vi "Teleop.vi"(10 "Match Info":T1={"Autonomous Elapsed Seconds"=0.0, "TeleOp Elapsed Seconds"=0.0, "Disabled Elapsed Seconds"=0.0, "Visited Autonomous"=FALSE, "Visited TeleOp"=FALSE, "Visited Disabled"=FALSE, "Autonomous Settings"={"Autonomous Style"=enum."Independent", "VI Refnum"=refnum}}, 11 "Call Context":T2) -> ()   [LabVIEW 2014]
doc: "This VI is called for each TeleOp packet received from the DS where the robot is not disabled. It is often used to read from the joysticks and update I/O or to update setpoints for timed control loops. It should complete and return within 20 milliseconds or it may miss DS packets."
uses:
  <vilib>/Rock Robotics/WPI/DriverStation/WPI_DriverStationDerivedRobotMode.ctl
  <vilib>/Rock Robotics/WPI/DriverStation/WPI_DriverStationMatch Info.ctl
  <vilib>/Rock Robotics/Network Tables/SD Read Boolean.vi
  <vilib>/Rock Robotics/Network Tables/SD Read Number.vi
  <vilib>/Rock Robotics/Network Tables/SD Write Numeric Array.vi
  1756_Code/General_VI/Global Var.vi
  <vilib>/Rock Robotics/Network Tables/SD Write Boolean Array.vi
panel:
  out "Sample Slider 0":dbl(slide) scale=0.0..5.0
  out "Sample Boolean 1":bool
  out "Sample Boolean 0":bool
  # "e"
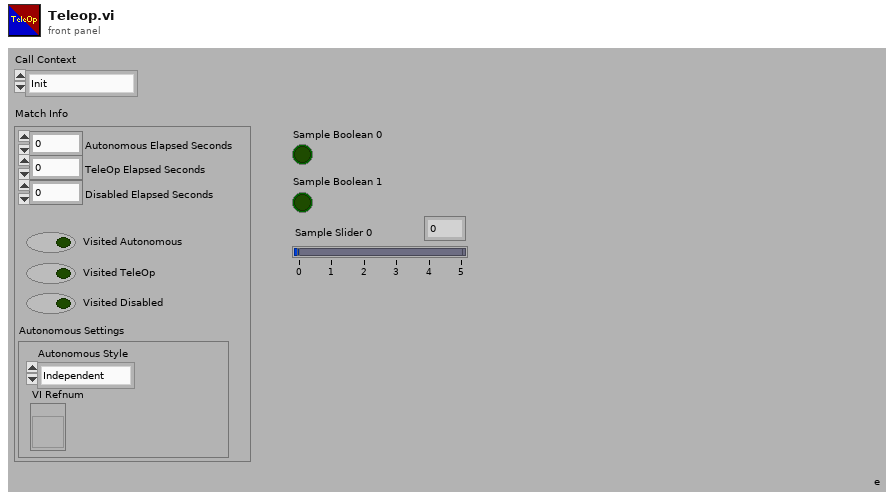
[diagram p1: front panel]
types:
  T1 = typedef "WPI_DriverStationMatch Info.ctl" = cluster{"Autonomous Elapsed Seconds":dbl, "TeleOp Elapsed Seconds":dbl, "Disabled Elapsed Seconds":dbl, "Visited Autonomous":bool, "Visited TeleOp":bool, "Visited Disabled":bool, "Autonomous Settings":cluster{"Autonomous Style":enum16{"Iterative", "Independent"}, "VI Refnum":refnum<vi>}}
  T2 = typedef "WPI_DriverStationDerivedRobotMode.ctl" = enum16{"Init", "Execute", "Stop"}
  T3 = typedef "WPI_JoystickDevRef.ctl" = cluster{"Device":T4}
  T4 = typedef "WPI_JoystickDeviceEnum.ctl" = enum16{"USB 0", "USB 1", "USB 2", "USB 3", "USB 4", "USB 5"}
  T5 = typedef "WPI_RobotDriveDevRef.ctl" = cluster{"DevStatus":errorcluster, "Motors[]":T6[], "Square Inputs":bool, "Max Output":dbl}
  T6 = typedef "WPI_MotorControlDeviceRef.ctl" = cluster{"DeviceStatus":errorcluster, "Type":T7, "PWM":cluster{"Controller":T8, "PWM Channel":T9, "DeadBand":T10}, "CAN":cluster{"Device Number":u8, "Control Mode":T11, "Semaphore":T12, "Max Vout":dbl, "TalonSRX Control Mode":T13}, "Invert":bool, "TransformRef":T14, "InvTransformRef":T14}
  T7 = typedef "WPI_MotorControlType.ctl" = enum16{"PWM", "CAN", "CANTalonSRX"}
  T8 = typedef "FPGA_TypedefDigitalModule.ctl" = enum16{"Controller 1"}
  T9 = typedef "FPGA_DIOPWMChannel.ctl" = enum8{"PWM 0", "PWM 1", "PWM 2", "PWM 3", "PWM 4", "PWM 5", "PWM 6", "PWM 7", "PWM 8", "PWM 9", "PWM MXP 0", "PWM MXP 1", "PWM MXP 2", "PWM MXP 3", "PWM MXP 4", "PWM MXP 5", "PWM MXP 6", "PWM MXP 7", "PWM MXP 8", "PWM MXP 9", "Invalid"}
  T10 = typedef "WPI_PWMDeadband.ctl" = cluster{"Name":string, "maxPositivePwm":i32, "minPositivePwm":i32, "centerPwm":i32, "maxNegativePwm":i32, "minNegativePwm":i32, "angularRange":u16}
  T11 = typedef "WPI_CANJaguar_ControlMode.ctl" = enum8{"Percent VBus", "Current", "Speed", "Position", "Voltage"}
  T12 = typedef "Semaphore RefNum" = refnum<k1>
  T13 = typedef "WPI_CANTalonSRX_APIControlMode.ctl" = enum8{"Percent VBus", "Speed", "Position", "Slave", "Unchanged / Invalid"}
  T14 = typedef "WPI_PWMTransform_ConPane.ctl" = refnum<vi>
  T15 = typedef "WPI_EncoderDevRef.ctl" = cluster{"DevStatus":errorcluster, "EncoderIndex":T16, "CounterIndex":T17, "DistancePerCount":dbl, "Decoding Type":T18}
  T16 = typedef "FPGA_EncoderIdx.ctl" = enum8{"Enc 0", "Enc 1", "Enc 2", "Enc 3", "Enc 4", "Enc 5", "Enc 6", "Enc 7", "Invalid"}
  T17 = typedef "FPGA_CounterCtrSystemIndex.ctl" = enum8{"Ctr 0", "Ctr 1", "Ctr 2", "Ctr 3", "Ctr 4", "Ctr 5", "Ctr 6", "Ctr 7", "Invalid"}
  T18 = typedef "WPI_EncoderType.ctl" = enum16{"1x", "2x", "4x"}
  T19 = typedef "WPI_SwitchDevRef.ctl" = cluster{"DevStatus":errorcluster, "DIO Channel":T20, "Controller":T8, "CntIndex":T17, "Normally Closed":bool}
  T20 = typedef "FPGA_DIOChannel.ctl" = enum8{"DIO 0", "DIO 1", "DIO 2", "DIO 3", "DIO 4", "DIO 5", "DIO 6", "DIO 7", "DIO 8", "DIO 9", "DIO MXP 0", "DIO MXP 1", "DIO MXP 2", "DIO MXP 3", "DIO MXP 4", "DIO MXP 5", "DIO MXP 6", "DIO MXP 7", "DIO MXP 8", "DIO MXP 9", "DIO MXP 10", "DIO MXP 11", "DIO MXP 12", "DIO MXP 13", "DIO MXP 14", "DIO MXP 15", "Invalid"}
  T21 = typedef "WPI_AnalogChannelDevRef.ctl" = cluster{"DevStatus":errorcluster, "Controller":T22, "Analog Channel":T23}
  T22 = typedef "FPGA_TypedefAnalogModule.ctl" = enum16{"Controller 1"}
  T23 = typedef "FPGA_AIChannel.ctl" = enum8{"AI 0", "AI 1", "AI 2", "AI 3", "AI MXP 0", "AI MXP 1", "AI MXP 2", "AI MXP 3", "Invalid"}
  T24 = typedef "IMUDevRef.ctl" = cluster{"DevStatus":errorcluster, "Gyro Address":u8, "Gyro Range":u8, "Mean Rates":cluster{"Xmo":dbl, "Ymo":dbl, "Zmo":dbl}, "StdDev Rates":cluster{"Xsdo":dbl, "Ysdo":dbl, "Zsdo":dbl}, "Fast":bool, "Reset":bool, "Accel Address":u8, "Accel Range":u8, "Accel Scale":cluster{"Xscale":dbl, "Yscale":dbl, "Zscale":dbl}, "Mag Address":u8, "Mag Range":u8, "G Sense":bool, "A Sense":bool, "M Sense":bool, "Accel Offset":cluster{"Xzero":dbl, "Yzero":dbl, "Zzero":dbl}, "Motion Thresh":dbl, "Mag Scale":cluster{"Xscale":dbl, "Yscale":dbl, "Zscale":dbl}, "Mag Offset":cluster{"Xzero":dbl, "Yzero":dbl, "Zzero":dbl}, "I2C Bus":T25, "Handle":i32, "Controller":T8, "Anomaly Thresh":dbl, "Local Mag":dbl}
  T25 = typedef "i2c_bus.ctl" = enum16{"I2C On-Board", "I2C MXP", "Invalid"}
  T26 = typedef "WPI_CompressorDevRef.ctl" = cluster{"DevStatus":errorcluster, "Pneumatics Control Module":u8}
  T27 = typedef "WPI_SolenoidDevRef.ctl" = cluster{"DevStatus":errorcluster, "Pneumatics Control Module":u8, "Forward Solenoid Channel":T28, "Reverse Solenoid Channel":T28}
  T28 = typedef "WPI_SolenoidChannel.ctl" = enum8{"Solenoid 0", "Solenoid 1", "Solenoid 2", "Solenoid 3", "Solenoid 4", "Solenoid 5", "Solenoid 6", "Solenoid 7", "Invalid"}
  T29 = cluster{"Joystick":cluster{"Drive_Joystick":T3, "Imp_Joystick":T3}, "Motor":cluster{"Left and Right Motors":T5, "Left_Intake":T6, "Right_Intake":T6, "Elevator_Lift":T6, "Elevator_Arm_Left":T6, "Elevator_Arm_Right":T6}, "Encoder":cluster{"Left_Drive_Speed":T15, "Auto_2_Tote":T19, "Auto_Cans":T19, "Auto_Cans_Delay":T19}, "Analog":cluster{"Tote_Detect_1":T21, "Tote_Detect_2":T21, "Ele_Pos_Yoyo":T21, "Auto_Switch":T21}, "IMU_Reft_Num":T24, "Pneumatics":cluster{"Compressor":T26, "Arm_Sol":T27, "Infeed_Pneu":T27, "Can_Tip_Flip":T27, "Can_Tip_Arm":T27, "Can_Door_Arm":T27, "Arm_Sol_Ext":T27}}
  T30 = cluster{"Left_Trigger":dbl, "Right_Trigger ":dbl, "Left_X":dbl, "Left_Y":dbl, "Right_X":dbl, "Right_Y":dbl}
  T31 = cluster{"A":bool, "B":bool, "X":bool, " Y":bool, "LB":bool, " RB":bool, "Left_Thumb_Button":bool, "Right_Thumb_Button":bool, "Back":bool, "Start":bool}
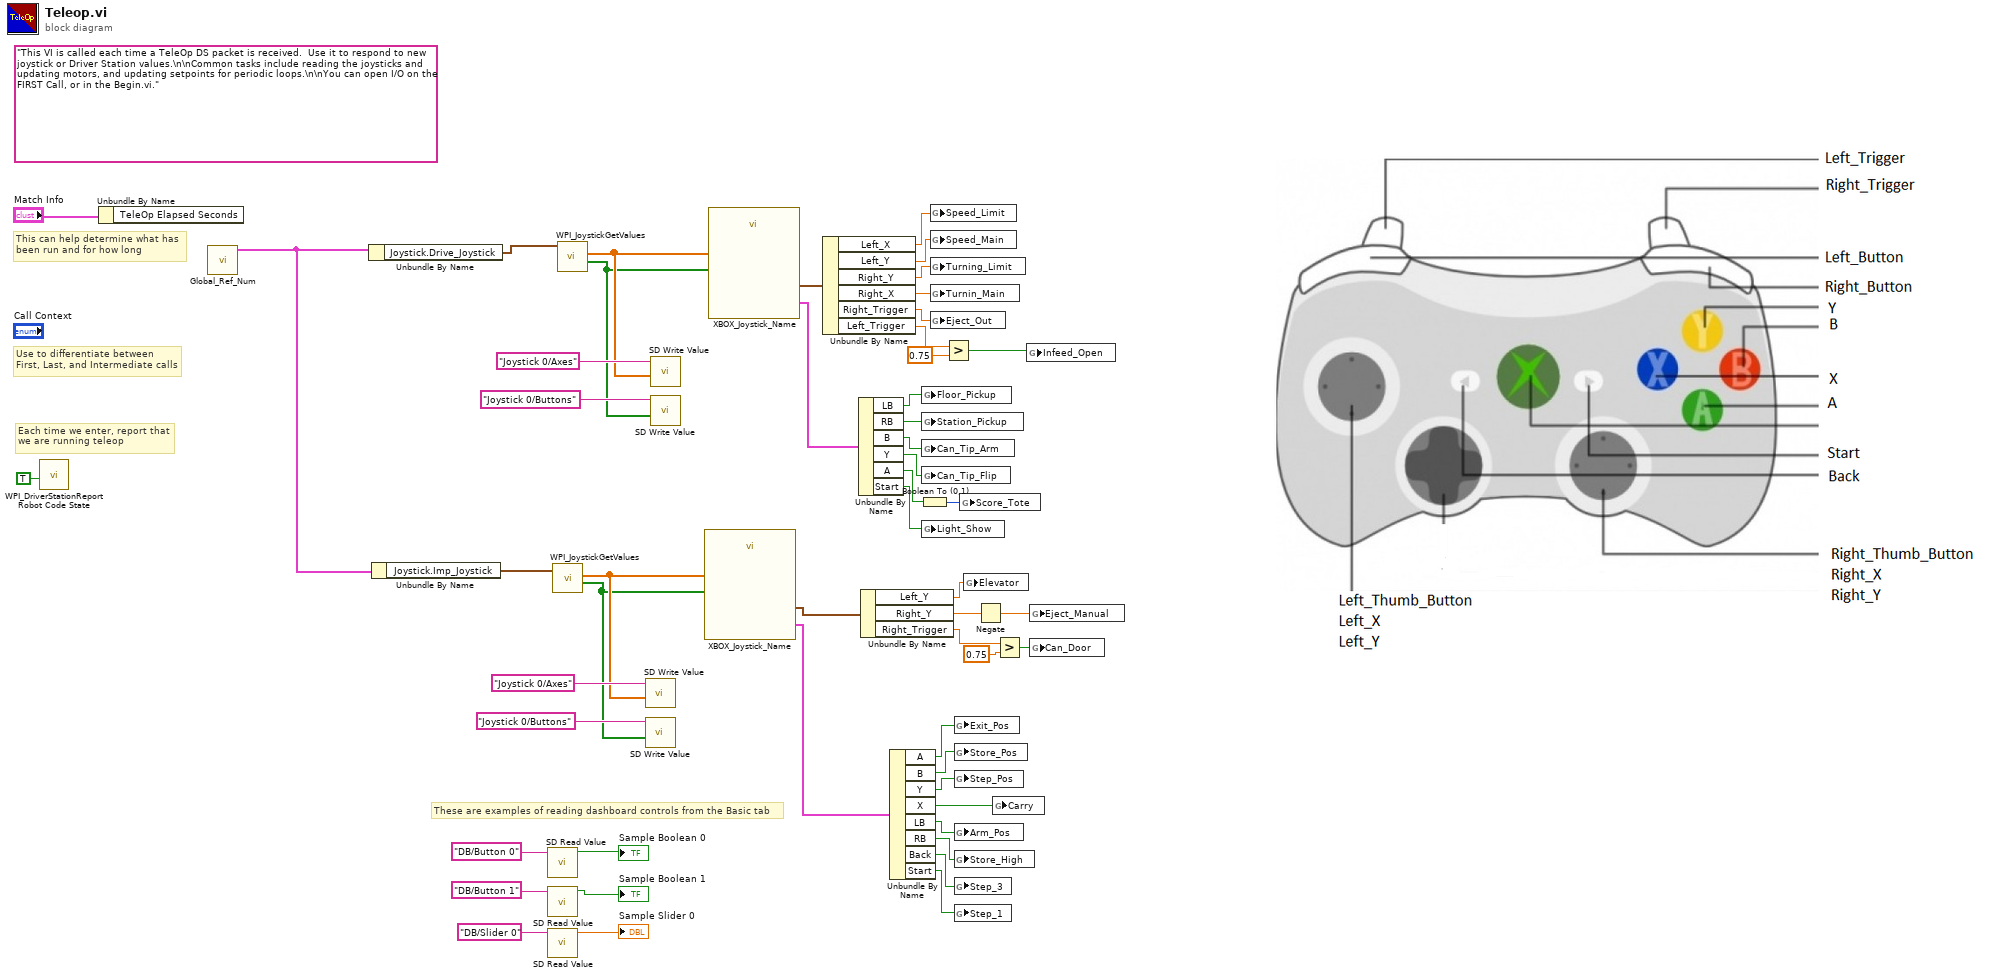
[diagram p0: block diagram]
diagram:
  (unwired) "This VI is called each time a TeleOp DS packet is received.  Use it to respond to new joystick or Driver Station values.\n\nCommon tasks include reading the joysticks and updating motors, and updating setpoints for periodic loops.\n\nYou can open I/O on the FIRST Call, or in the Begin.vi."
  # "These are examples of reading dashboard controls from the Basic tab"
  # "Each time we enter, report that\nwe are running teleop"
  # "Use to differentiate between\nFirst, Last, and Intermediate calls"
  # "This can help determine what has\nbeen run and for how long"
  n1 = call <vilib>:"WPI_DriverStationReport Robot Code State.vi"("TeleOp"=TRUE ("Autonomous")) -> ()  [unwired: 10 in, 1 out]
  n2 = Unbundle By Name("Match Info") -> ()  [unwired: 1 out]
  n3 = call "Global_Ref_Num.vi"() -> ("Ref_Num"=w24:T29)  [unwired: 10 in]
  n4 = Unbundle By Name(w24) -> ("Joystick.Drive_Joystick"=w26:T3)
  n5 = Unbundle By Name(w24) -> ("Joystick.Imp_Joystick"=w25:T3)
  n6 = call-poly <vilib>:"SD Read Value.vi"("Name"="DB/Button 0" ("refnum name")) -> ("Boolean"=→"Sample Boolean 0":bool)  [unwired: 8 in, 2 out]
  n7 = call-poly <vilib>:"SD Read Value.vi"("Name"="DB/Button 1" ("refnum name")) -> ("Boolean"=→"Sample Boolean 1":bool)  [unwired: 8 in, 2 out]
  n8 = call-poly <vilib>:"SD Read Value.vi"("Name"="DB/Slider 0" ("refnum name")) -> ("Numeric"=→"Sample Slider 0":dbl)  [unwired: 8 in, 2 out]
  n9 = call <vilib>:"WPI_JoystickGetValues.vi"("JoystickDevRef"=w25) -> ("Buttons"=w29:bool[], "Axes"=w30:dbl[])  [unwired: 6 in, 3 out]
  n10 = call <vilib>:"WPI_JoystickGetValues.vi"("JoystickDevRef"=w26) -> ("Buttons"=w41:bool[], "Axes"=w42:dbl[])  [unwired: 6 in, 3 out]
  n11 = call-poly <vilib>:"SD Write Value.vi"("Numeric Array"=w30, "Name"="Joystick 0/Axes") -> ()  [unwired: 8 in, 2 out]
  n12 = call-poly <vilib>:"SD Write Value.vi"("Boolean Array"=w29, "Name"="Joystick 0/Buttons") -> ()  [unwired: 8 in, 2 out]
  n13 = call-poly <vilib>:"SD Write Value.vi"("Numeric Array"=w42, "Name"="Joystick 0/Axes") -> ()  [unwired: 8 in, 2 out]
  n14 = call-poly <vilib>:"SD Write Value.vi"("Boolean Array"=w41, "Name"="Joystick 0/Buttons") -> ()  [unwired: 8 in, 2 out]
  n15 = call "XBOX_Joystick_Name.vi"("Buttons"=w29, "Axes"=w30) -> ("Named_Joystick"=w28:T30, "Named_Buttons"=w27:T31)  [unwired: 8 in]
  n16 = call "XBOX_Joystick_Name.vi"("Buttons"=w41, "Axes"=w42) -> ("Named_Joystick"=w40:T30, "Named_Buttons"=w35:T31)  [unwired: 8 in]
  n17 = Unbundle By Name(w40) -> ("Left_X"=w39:dbl, "Left_Y"=w38:dbl, "Right_Y"=w37:dbl, "Right_X"=w36:dbl, "Right_Trigger"=w23:dbl, "Left_Trigger"=w10:dbl)
  n18 = Unbundle By Name(w35) -> ("LB"=w34:bool, "RB"=w33:bool, "B"=w15:bool, "Y"=w14:bool, "A"=w12:bool, "Start"=w5:bool)
  n19 = Unbundle By Name(w28) -> ("Left_Y"=w22:dbl, "Right_Y"=w7:dbl, "Right_Trigger"=w3:dbl)
  n20 = Unbundle By Name(w27) -> ("A"=w21:bool, "B"=w20:bool, "Y"=w18:bool, "X"=w17:bool, "LB"=w19:bool, "RB"=w1:bool, "Back"=w16:bool, "Start"=w13:bool)
  n21 = Boolean To (0,1)(Boolean=w12) -> (0, 1=w11:i16)
  n22 = global write "Global Var.vi" "Floor_Pickup"(w34) -> ()
  n23 = global write "Global Var.vi" "Station_Pickup"(w33) -> ()
  n24 = global write "Global Var.vi" "Can_Tip_Arm"(w15) -> ()
  n25 = global write "Global Var.vi" "Can_Tip_Flip"(w14) -> ()
  n26 = global write "Global Var.vi" "Light_Show"(w5) -> ()
  n27 = global write "Global Var.vi" "Speed_Limit"(w39) -> ()
  n28 = global write "Global Var.vi" "Speed_Main"(w38) -> ()
  n29 = global write "Global Var.vi" "Turning_Limit"(w37) -> ()
  n30 = global write "Global Var.vi" "Turnin_Main"(w36) -> ()
  n31 = global write "Global Var.vi" "Eject_Out"(w23) -> ()
  n32 = Greater?(x=w10, y=0.75) -> (0:w8:bool)
  n33 = global write "Global Var.vi" "Exit_Pos"(w21) -> ()
  n34 = global write "Global Var.vi" "Store_Pos"(w20) -> ()
  n35 = global write "Global Var.vi" "Step_Pos"(w18) -> ()
  n36 = global write "Global Var.vi" "Arm_Pos"(w19) -> ()
  n37 = global write "Global Var.vi" "Store_High"(w1) -> ()
  n38 = global write "Global Var.vi" "Step_3"(w16) -> ()
  n39 = global write "Global Var.vi" "Step_1"(w13) -> ()
  n40 = global write "Global Var.vi" "Score_Tote"(w11) -> ()
  n41 = global write "Global Var.vi" "Elevator"(w22) -> ()
  n42 = Negate(x=w7) -> (-x=w6:dbl)
  n43 = global write "Global Var.vi" "Carry"(w17) -> ()
  n44 = Greater?(x=w3, y=0.75) -> (0:w2:bool)
  n45 = global write "Global Var.vi" "Infeed_Open"(w8) -> ()
  n46 = global write "Global Var.vi" "Eject_Manual"(w6) -> ()
  n47 = global write "Global Var.vi" "Can_Door"(w2) -> ()
